vi "Software Update HCC Get Stations and IDs.vi"(8 "Error In":errorcluster, 10 "Station Location (Index)":u32, 11 "Stations and Board IDs":path) -> (0 "Error Out":errorcluster, 1 "Updated Input":string[](array[string]), 2 "Station index":u32, 3 "List of Stations and Board IDs":string[][](array[string]), 4 "Station Name":string)   [LabVIEW 2016]
uses:
  <vilib>/Utility/file.llb/Read Delimited Spreadsheet (string).vi
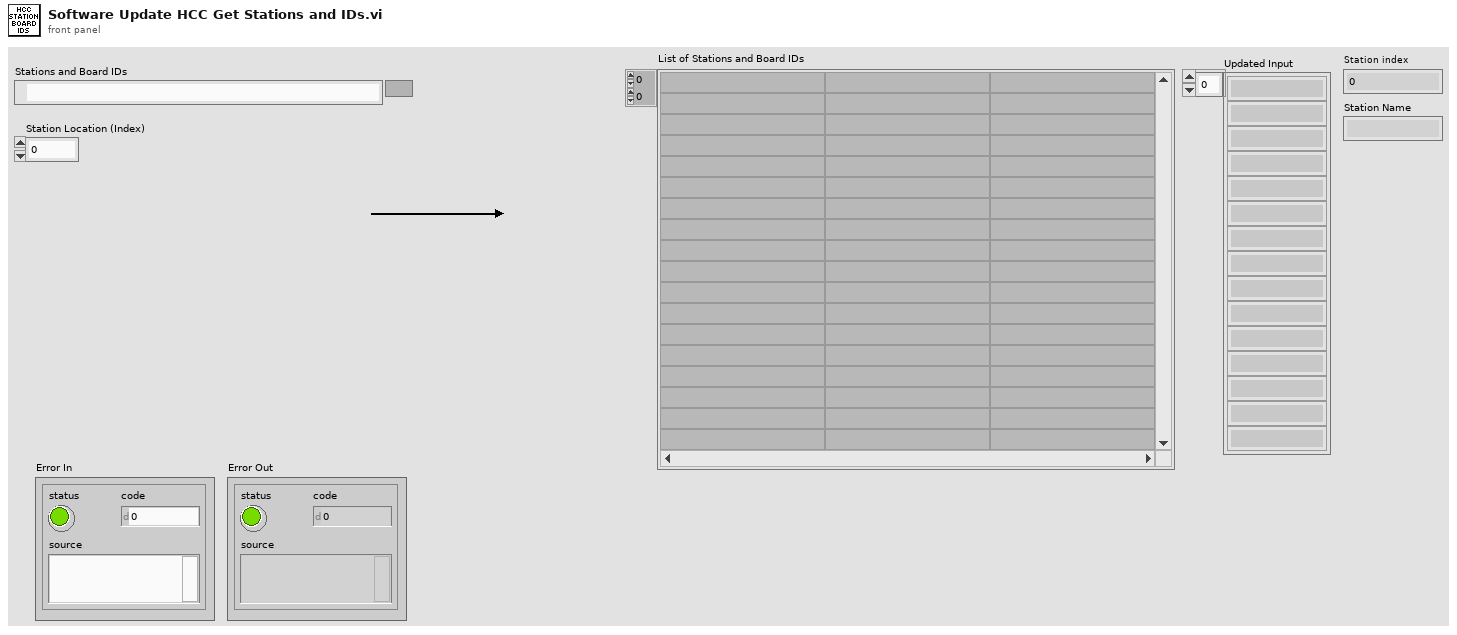
[diagram p1: front panel]
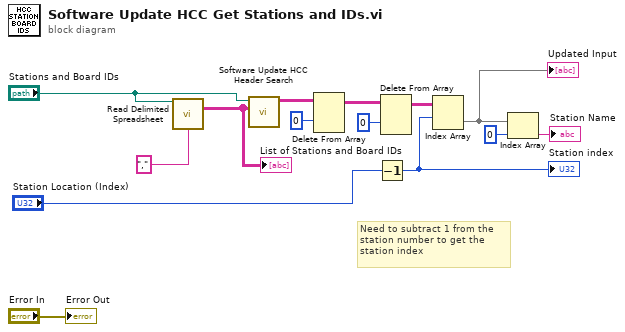
[diagram p0: block diagram]
diagram:
  # "Need to subtract 1 from the \nstation number to get the \nstation index"
  n1 = call-poly <vilib>:"Read Delimited Spreadsheet.vi"("file path (dialog if empty)"="Stations and Board IDs", "delimiter (\\t)"="," ("delimiter (\\t)")) -> ("all rows"=w13:string[][])  [unwired: 8 in, 5 out]
  "List of Stations and Board IDs" <- w13
  n2 = call "Software Update HCC Header Search.vi"("Input Data"=w13, "Station And Board ID Paths"="Stations and Board IDs") -> ("Updated Input"=w10:string[][])  [unwired: 9 in]
  n3 = Delete From Array(array=w10, index (row)=0) -> (array with subset deleted=w6:string[][])  [unwired: 2 in, 1 out]
  n4 = Decrement(x="Station Location (Index)") -> (x-1=w11:u32)
  "Station index" <- w11
  n5 = Delete From Array(array=w6, index (row)=0) -> (array with subset deleted=w8:string[][])  [unwired: 2 in, 1 out]
  n6 = Index Array(array=w8, index (row)=w11) -> (element=w3:string[])  [unwired: 1 in]
  "Updated Input" <- w3
  n7 = Index Array(array=w3, index=0) -> (element=→"Station Name":string)
  "Error Out" <- "Error In"
